vi "Initialize FGEN.vi"(8 "error in (no error)":errorcluster, 10 "FGEN Settings":T1, 11 "FGEN Resource In":refnum<k15>) -> (0 "error out":errorcluster, 2 "Total Wfm Duration (s)":dbl, 3 "FGEN Resource Out":refnum<k15>)   [LabVIEW 2025]
uses:
  <instrlib>/niFgen/niFgen.llb/niFgen Output Mode.ctl
  <instrlib>/niFgen/niFgen.llb/niFgen Trigger Mode.ctl
  <instrlib>/niFgen/niFgen.llb/niFgen Disable Start Trigger.vi
  <instrlib>/niFgen/niFgen.llb/niFgen Create Waveform (WDT).vi
  <vilib>/Waveform/WDTOps.llb/WDT Waveform Duration DBL.vi
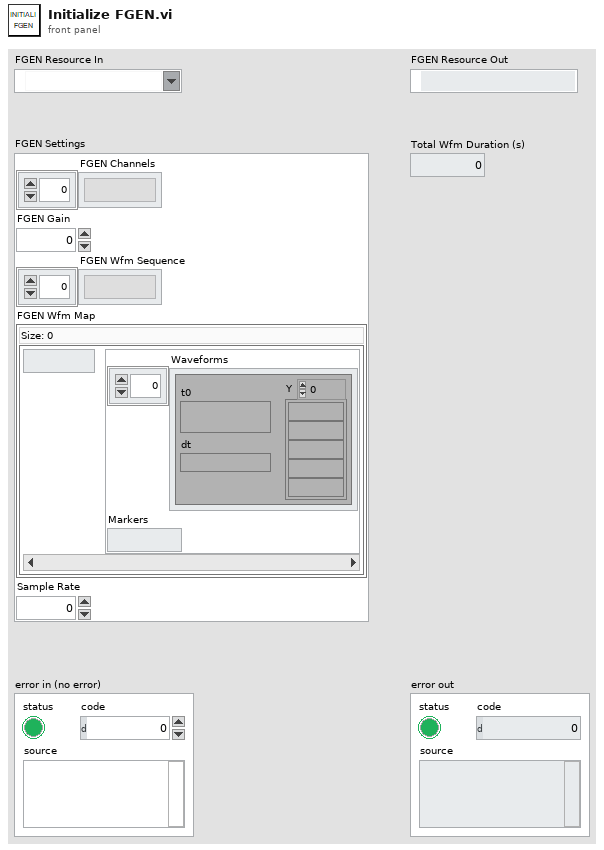
[diagram p1: front panel]
types:
  T1 = cluster{"FGEN Channels":string[], "FGEN Gain":dbl, "FGEN Wfm Sequence":string[], "FGEN Wfm Map":map{string, cluster{"Waveforms":waveform(dbl)[], "Markers":i32}}, "Sample Rate":dbl}
  T2 = typedef "niFgen Trigger Mode.ctl" = i32
  T3 = typedef "niFgen Output Mode.ctl" = u32
  T4 = map{string, cluster{"Waveforms":waveform(dbl)[], "Markers":i32}}
  T5 = map{string, cluster{"Markers":i32, "Waveform Handle":i32}}
  T6 = cluster{"Waveforms":waveform(dbl)[], "Markers":i32}
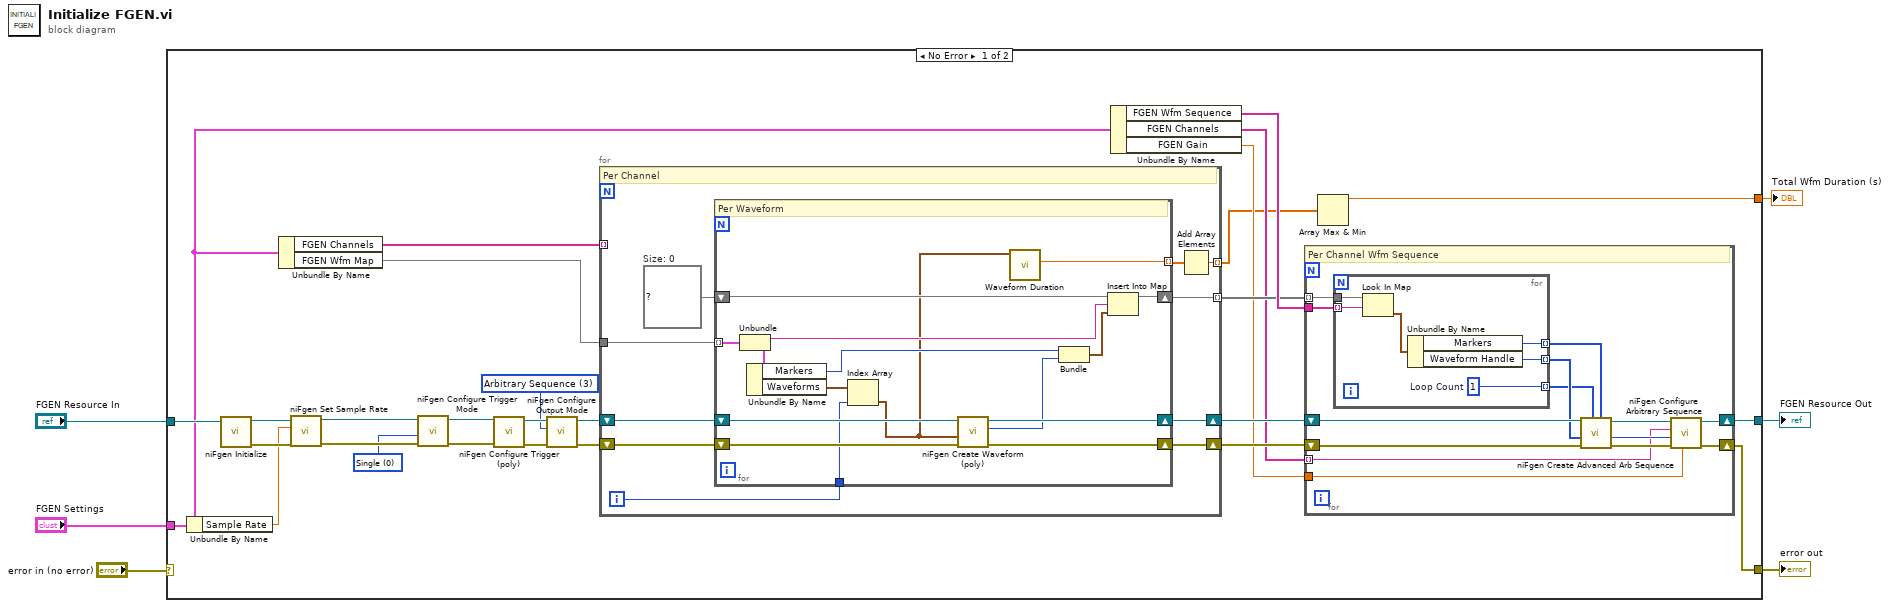
[diagram p0: block diagram]
diagram:
  n1 = case shown="No Error" "error in (no error)" {
    selector: "error in (no error)" -> [_ w81]
    tunnel: [w10 w81] -> w6
    tunnel: "FGEN Resource In" -> [w33 w80]
    tunnel: "FGEN Settings" -> [w32 _]
    tunnel: [w31 w80] -> w2
    tunnel: [w7 _] -> w1
    frame No Error {
      w9 = T2 0 items=["Single", "Continuous", "Stepped", "Burst"] ("Trigger Mode (default: 1=continuous)")
      w22 = T3 3 items=["Standard Function", "Frequency List", "Arbitrary Waveform", "Arbitrary Sequence", "Script"] ("Output Mode")
      n2 = Unbundle By Name(w32) -> ("Sample Rate"=w19:dbl)
      n3 = call <instrlib>:"niFgen Initialize.vi"("Resource Name"=w33) -> ("error out"=w29:errorcluster, "Instrument Handle Out"=w30:refnum<k15>)  [unwired: 9 in]
      n4 = Unbundle By Name(w32) -> ("FGEN Channels"=w17:string[], "FGEN Wfm Map"=w18:T4)
      n5 = call <instrlib>:"niFgen Set Sample Rate.vi"("error in (no error)"=w29, "Sample Rate (Samp/s)"=w19, "Instrument Handle"=w30) -> ("error out"=w27:errorcluster, "Instrument Handle Out"=w28:refnum<k15>)  [unwired: 7 in]
      n6 = call <instrlib>:"niFgen Configure Trigger Mode.vi"("error in (no error)"=w27, "Trigger Mode (default: 1=continuous)"=w9, "Instrument Handle"=w28) -> ("error out"=w25:errorcluster, "Instrument Handle Out"=w26:refnum<k15>)  [unwired: 7 in]
      n7 = call-poly <instrlib>:"niFgen Configure Trigger (poly).vi"("error in (no error)"=w25, "Instrument Handle"=w26) -> ("error out"=w23:errorcluster, "Instrument Handle Out"=w24:refnum<k15>)  [unwired: 8 in]
      n8 = call <instrlib>:"niFgen Configure Output Mode.vi"("error in (no error)"=w23, "Output Mode (default: 0=Standard Function)"=w22, "Instrument Handle"=w24) -> ("error out"=w20:errorcluster, "Instrument Handle Out"=w21:refnum<k15>)  [unwired: 6 in]
      n9 = for {
        tunnel: w18 -> [w59]
        tunnel: w17 -> [_] mode=indexing
        shift-right: [w61] -> w13
        shift-left: w20 -> [w62]
        shift-right: [w60] -> w14
        shift-left: w21 -> [w63]
        tunnel: [w56] -> w15 mode=indexing
        tunnel: [w54] -> w8 mode=indexing
        i -> [w58]
        w57 = T5 {}  # Size: 0
        # "Per Channel"
        n10 = for {
          shift-right: [w78] -> w61
          shift-left: w62 -> [w76]
          shift-right: [w79] -> w60
          shift-left: w63 -> [w77]
          tunnel: w59 -> [w75] mode=indexing
          tunnel: w58 -> [w72]
          shift-right: [w66] -> w56
          shift-left: w57 -> [w69]
          tunnel: [w64] -> w55 mode=indexing
          # "Per Waveform"
          n11 = Unbundle(w75) -> (w68:string, "output cluster"=w74:T6)
          n12 = Unbundle By Name(w74) -> ("Markers"=w71:i32, "Waveforms"=w73:waveform(dbl)[])
          n13 = Index Array(array=w73, index=w72) -> (element=w65:waveform(dbl))
          n14 = call-poly <instrlib>:"niFgen Create Waveform (poly).vi"("error in (no error)"=w76, "Waveform"=w65, "Instrument Handle"=w77) -> ("error out"=w78:errorcluster, "Waveform Handle"=w70:i32, "Instrument Handle Out"=w79:refnum<k15>)  [unwired: 6 in]
          n15 = call-poly <vilib>:"Waveform Duration.vi"("waveform in"=w65) -> ("duration"=w64:dbl)  [unwired: 8 in, 2 out]
          n16 = Bundle("Markers"=w71, "Waveform Handle"=w70) -> (w67:cluster{"Markers":i32, "Waveform Handle":i32})  [unwired: 1 in]
          n17 = Insert Into Map(map in=w69, key=w68, value=w67) -> (map out=w66:T5)  [unwired: 2 out]
        }
        n18 = Add Array Elements(numeric array=w55) -> (sum=w54:dbl)
      }
      n19 = Unbundle By Name(w32) -> ("FGEN Wfm Sequence"=w16:string[], "FGEN Channels"=w12:string[], "FGEN Gain"=w11:dbl)
      n20 = for {
        tunnel: w16 -> [w47]
        tunnel: w15 -> [w46] mode=indexing
        shift-right: [w37] -> w31
        shift-left: w14 -> [w45]
        shift-right: [w39] -> w10
        shift-left: w13 -> [w40]
        tunnel: w12 -> [w35] mode=indexing
        tunnel: w11 -> [w34]
        # "Per Channel Wfm Sequence"
        n21 = for {
          tunnel: w47 -> [w53] mode=indexing
          tunnel: w46 -> [w52]
          tunnel: [w50] -> w44 mode=indexing
          tunnel: [w49] -> w43 mode=indexing
          tunnel: [w48] -> w42 mode=indexing
          w48 = 1  # Loop Count
          n22 = Look In Map(map=w52, key=w53) -> (value=w51:cluster{"Markers":i32, "Waveform Handle":i32})  [unwired: 1 in, 1 out]
          n23 = Unbundle By Name(w51) -> ("Markers"=w49:i32, "Waveform Handle"=w50:i32)
        }
        n24 = call <instrlib>:"niFgen Create Advanced Arb Sequence.vi"("Marker Location Array"=w43, "Loop Counts Array"=w42, "error in (no error)"=w40, "Waveform Handles Array"=w44, "Instrument Handle"=w45) -> ("error out"=w41:errorcluster, "Sequence Handle"=w36:i32, "Instrument Handle Out"=w38:refnum<k15>)  [unwired: 3 in, 1 out]
        n25 = call <instrlib>:"niFgen Configure Arbitrary Sequence.vi"("Gain"=w34, "error in (no error)"=w41, "Sequence Handle"=w36, "Channel Name"=w35, "Instrument Handle"=w38) -> ("error out"=w39:errorcluster, "Instrument Handle Out"=w37:refnum<k15>)  [unwired: 5 in]
      }
      n26 = Array Max & Min(array=w8) -> (max value=w7:dbl)  [unwired: 3 out]
    }
    frame Error {
    }
  }
  "error out" <- w6
  "FGEN Resource Out" <- w2
  "Total Wfm Duration (s)" <- w1
